vi "PixelsPerCharacter.vi"(8 "error in (no error)":errorcluster, 11 "Code39 in":refnum<class "Code39.lvclass">) -> (0 "error out":errorcluster, 2 "Pixels per Character":u8, 3 "Code39 out":refnum<class "Code39.lvclass">)   [LabVIEW 2013, in "BarCodes.lvlib" / "Code39.lvclass"]
uses:
  Code39.lvclass
  Code39.lvclass/Code39.ctl
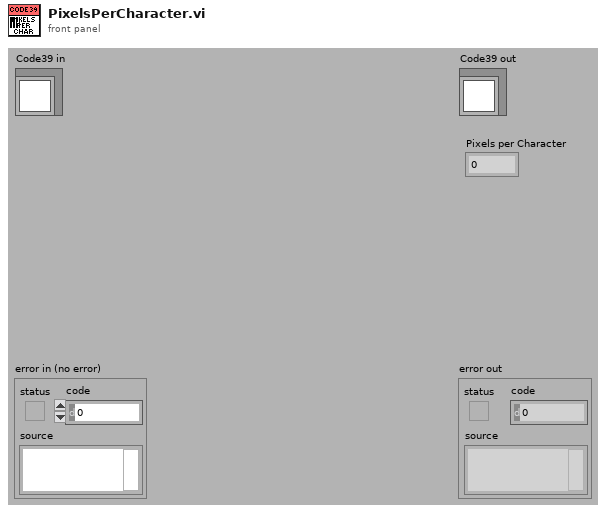
[diagram p1: front panel]
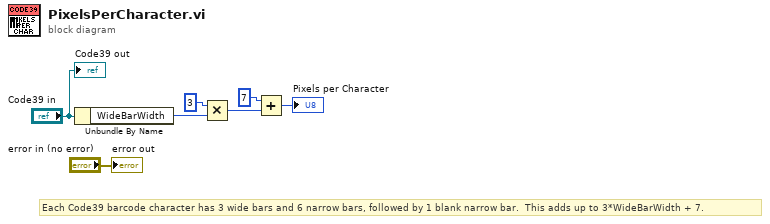
[diagram p0: block diagram]
diagram:
  # "Each Code39 barcode character has 3 wide bars and 6 narrow bars, followed by 1 blank narrow bar.  This adds up to 3*WideBarWidth + 7."
  n1 = Unbundle By Name("Code39 in") -> ("WideBarWidth"=w2:u8)
  n2 = Multiply(x=u8 3, y=w2) -> (x*y=w4:u8)
  n3 = Add(x=u8 7, y=w4) -> (x+y=→"Pixels per Character":u8)
  "error out" <- "error in (no error)"
  "Code39 out" <- "Code39 in"
